vi "RemoveWhitespaces.vi"(8 "error in (no error)":errorcluster, 11 "Array In":string[](array[string])=["r", "tr", "5", "", "56", "rt"]) -> (0 "error out":errorcluster, 3 "Array removing empty space":string[](array[string]))   [LabVIEW 2014, in "TableLogger_CSV_Actor.lvlib" / "TableLogger_CSV_Actor.lvclass"]
uses:
  TableLogger_CSV_Actor.lvclass
panel:
  # "Connector Pane"
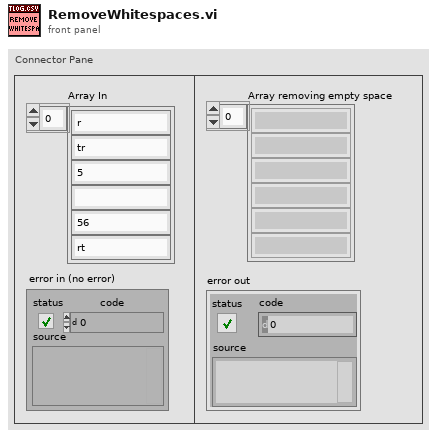
[diagram p1: front panel]
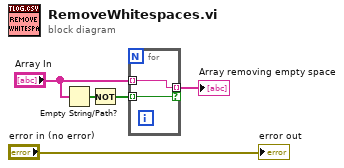
[diagram p0: block diagram]
diagram:
  n1 = Empty String/Path?(string/path="Array In") -> (empty?=w4:bool[])
  n2 = Not(x=w4) -> (.not. x?=w3:bool[])
  n3 = for {
    tunnel: w3 -> [w7] mode=indexing
    tunnel: [w6] -> w1 mode=indexing if=w7
    tunnel: "Array In" -> [w6] mode=indexing
  }
  "Array removing empty space" <- w1
  "error out" <- "error in (no error)"
